vi "ClassAppData.Init.vi"(8 "error in (no error)":errorcluster, 9 "Module Name":string, 10 "App Data Dir":path, 11 "Class - App Data in":refnum<class "Class.AppData.lvclass">) -> (0 "error out":errorcluster, 2 "File":path, 3 "Class - App Data out":refnum<class "Class.AppData.lvclass">)   [LabVIEW 2024, in "EQMF.lvlib" / "Config Utils.lvlib" / "Class.AppData.lvclass"]
doc: "<B>AppData Class:</B>\nThe AppData class keeps track of a library of data items that are used by an application. These data items have a name (text string) and value that can be any data type. \n\n<B>AppData.Init VI:</B>\nThis VI reads the data library items from a binary file at the location specified by the inputs App Data Dir and Module Name. The file path will be \"<App Data Dir>\\<Module Name>.dat\"\nThis VI is meant to be used at the application launch to restore the data library to the state it was in when the application last exited. The library items will be available when other call member VIs are called to update, retrieve, or delete them.\n\nIf the data file does not exist, then this VI will output an error."
uses:
  Class.AppData.lvclass
  Class.AppData.lvclass/Class.AppData.ctl
  Files/File Utils.lvlib
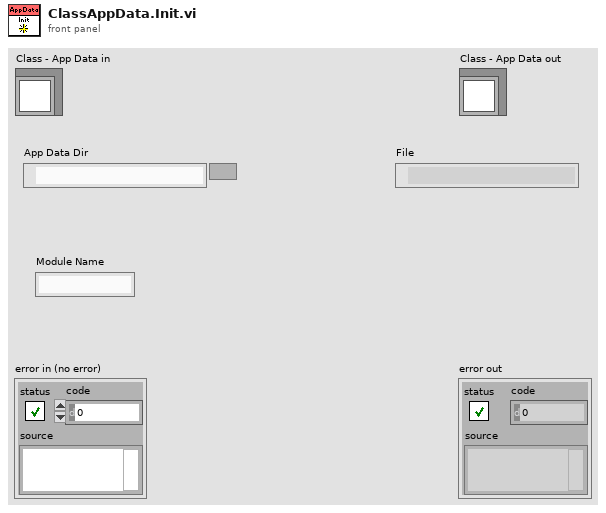
[diagram p1: front panel]
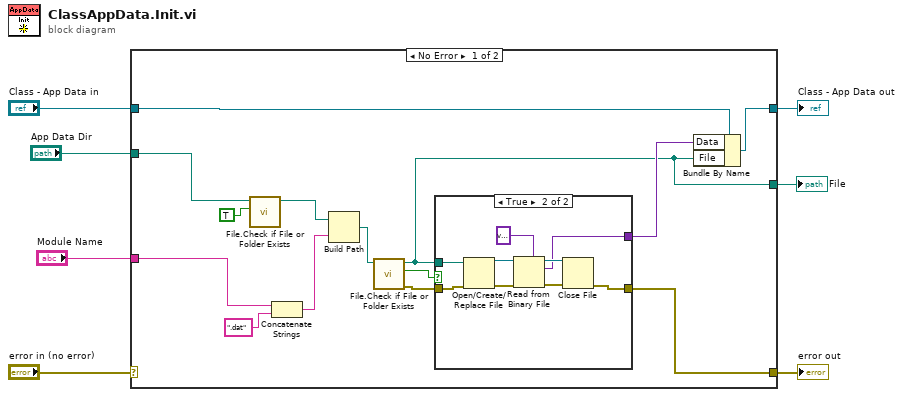
[diagram p0: block diagram]
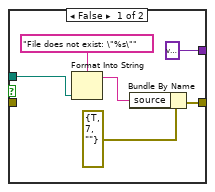
[diagram p2: hidden frame]
diagram:
  n1 = case shown="No Error" "error in (no error)" {
    selector: "error in (no error)" -> [_ w38]
    tunnel: [w8 w38] -> w6
    tunnel: [w21 w37] -> w4
    tunnel: "Class - App Data in" -> [w20 w37]
    tunnel: [w16 _] -> w3
    tunnel: "App Data Dir" -> [w13 _]
    tunnel: "Module Name" -> [w12 _]
    frame No Error {
      n2 = call "File.Check if File or Folder Exists.vi"("Create Dir if does not Exist"=TRUE, "Path"=w13) -> ("Dup Path"=w15:path)  [unwired: 5 in, 4 out]
      n3 = Concatenate Strings(w12, ".dat" ("string")) -> (w10:string)
      n4 = Build Path(base path=w15, name or relative path=w10) -> (appended path=w19:path)
      n5 = call "File.Check if File or Folder Exists.vi"("Path"=w19) -> ("error out"=w9:errorcluster, "Exists"=w18:bool, "Dup Path"=w16:path)  [unwired: 6 in, 2 out]
      n6 = case shown="True" w18 {
        tunnel: w16 -> [w25 w31]
        tunnel: [variant w30] -> w17
        tunnel: w9 -> [_ w29]
        tunnel: [w22 w28] -> w8
        frame False {
          n7 = Format Into String(format string="File does not exist: \"%s\"", w25) -> (resulting string=w23:string)  [unwired: 2 in, 1 out]
          n8 = Bundle By Name(cluster=errorcluster {"status"=TRUE, "code"=7, "source"=""} ("error constant"), "source"=w23) -> (w22:errorcluster)
        }
        frame True {
          n9 = Open/Create/Replace File(file path (use dialog)=w31, error in=w29) -> (refnum out=w33:refnum<file>, error out=w32:errorcluster)  [unwired: 4 in, 1 out]
          n10 = Read from Binary File(5:variant, 8:w32, 11:w33) -> (0:w36:errorcluster, 2:w30:variant, 3:w35:refnum<file>)  [unwired: 3 in, 1 out]
          n11 = Close File(refnum=w35, error in=w36) -> (error out=w28:errorcluster)  [unwired: 1 out]
        }
      }
      n12 = Bundle By Name(cluster=w20, "Data"=w17, "File"=w16) -> (w21:refnum<class "Class.AppData.lvclass">)
    }
    frame Error {
    }
  }
  "error out" <- w6
  "Class - App Data out" <- w4
  "File" <- w3
